vi "Data Access.vi"(8 "error in (no error)":errorcluster, 10 "Data Access Handler":refnum<class "Data Access Handler.lvclass">, 11 "Display Pop Up Msg in":refnum<class "Display Pop Up Msg.lvclass">) -> (0 "error out":errorcluster, 3 "Display Pop Up Msg Msg out":refnum<class "Display Pop Up Msg.lvclass">)   [LabVIEW 2020, in "Msg.lvlib" / "Display Pop Up Msg.lvclass"]
doc: "Expose class private data to the front panel while letting the Data Access Handler class act on the data."
uses:
  Display Pop Up Msg.lvclass
  C:/Current projects/WS/Framework/Framework/Messages/Msg/Flex Msg/Flex Msg.lvclass
  Flex Msg/Data Access Handlers/Data Access Handler/Data Access Handler.lvclass
  Display Pop Up Msg.lvclass/Display Pop Up Msg.ctl
panel:
  in  "Display time out":i32=-1
  in  "Pause?":bool=TRUE
  in  "Content":string
  in  "Header":string
  in  "Cancel":bool
  in  "OK":bool
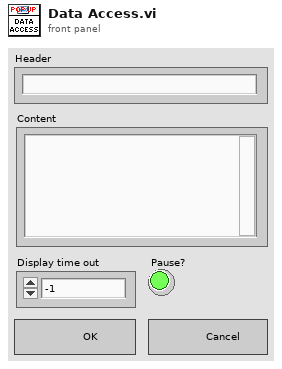
[diagram p1: front panel]
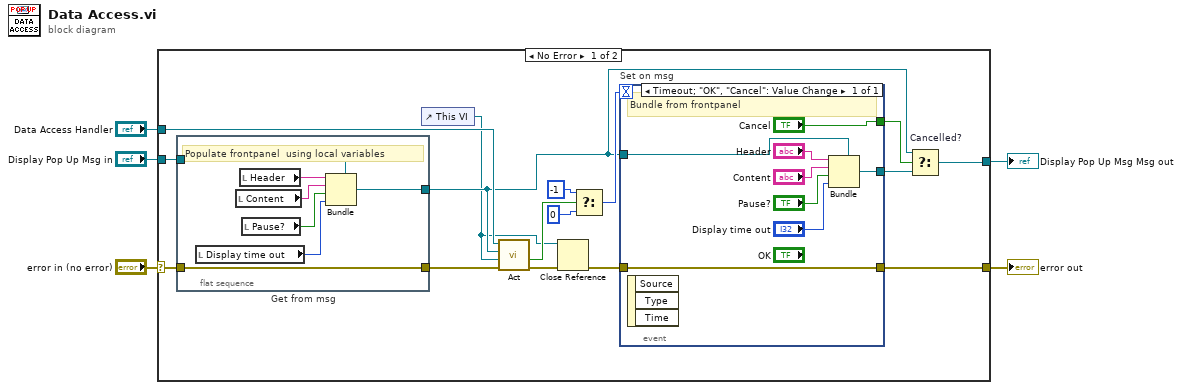
[diagram p0: block diagram]
diagram:
  n1 = case shown="No Error" "error in (no error)" {
    selector: "error in (no error)" -> [w21 w38]
    tunnel: [w14 w38] -> w4
    tunnel: [w9 w37] -> w2
    tunnel: "Display Pop Up Msg in" -> [w12 w37]
    tunnel: "Data Access Handler" -> [w20 _]
    frame No Error {
      n2 = flat-sequence "Get from msg" {
        tunnel: w21 -> [w36]
        tunnel: [w34] -> w7
        tunnel: w12 -> [w35]
        tunnel: [w36] -> w19
        frame #0 {
          # "Populate frontpanel  using local variables"
          n3 = local read "Display time out"() -> (w30:i32)
          n4 = local read "Content"() -> (w32:string)
          n5 = local read "Header"() -> (w33:string)
          n6 = local read "Pause?"() -> (w31:bool)
          n7 = Bundle(cluster=w35, w33, w32, w31, w30) -> (w34:refnum<class "Display Pop Up Msg.lvclass">)
        }
      }
      n8 = control-ref of="This VI"() -> (w6:refnum<vi>)
      n9 = call-dynamic "Act.vi"("error in (no error)"=w19, "VI Refnum in"=w6, "Flex Msg type"=w7, "Data Access Handler in"=w20) -> ("error out"=w11:errorcluster, "Await user action?"=w18:bool)  [unwired: 5 in, 1 out]
      n10 = Close Reference(reference=w6, error in (no error)=w11) -> (error out=w13:errorcluster)
      n11 = Select(t=-1, s=w18, f=0 ("t")) -> (s? t:f=w15:i32)
      n12 = event "Set on msg" shown="[0] Timeout;  \"OK\", \"Cancel\": Value Change" {
        selector: _ -> [_]
        dyn-events: _ -> [_]
        timeout: w15 -> [_]
        tunnel: [w29] -> w14
        tunnel: w13 -> [w29]
        tunnel: ["Cancel"] -> w10
        tunnel: [w26] -> w8
        tunnel: w7 -> [w28]
        event Timeout; "OK", "Cancel": Value Change {
          # "Bundle from frontpanel"
          n13 = event-data() -> ()  [unwired: 1 in, 3 out]
          n14 = Bundle(cluster=w28, "Header", "Content", "Pause?", "Display time out") -> (w26:refnum<class "Display Pop Up Msg.lvclass">)
        }
      }
      n15 = Select "Cancelled?"(t=w7, s=w10, f=w8) -> (s? t:f=w9:refnum<class "Display Pop Up Msg.lvclass">)
    }
    frame Error {
    }
  }
  "error out" <- w4
  "Display Pop Up Msg Msg out" <- w2
